vi "coolUI.vi"(11 "CoolDisplay.lvclass":refnum<class "CoolDisplay.lvclass">) -> ()   [LabVIEW 2018, in "CoolDisplay.lvclass"]
uses:
  CoolDisplay.lvclass
panel:
  out "Waveform Chart":cluster{"Humidity":dbl, "Pressure":dbl}(graph)
  out "Temperature":dbl(slide) scale=0.0..10.0
  out "error out":errorcluster
  in  "error in (no error)":errorcluster
  # "Cool Display"
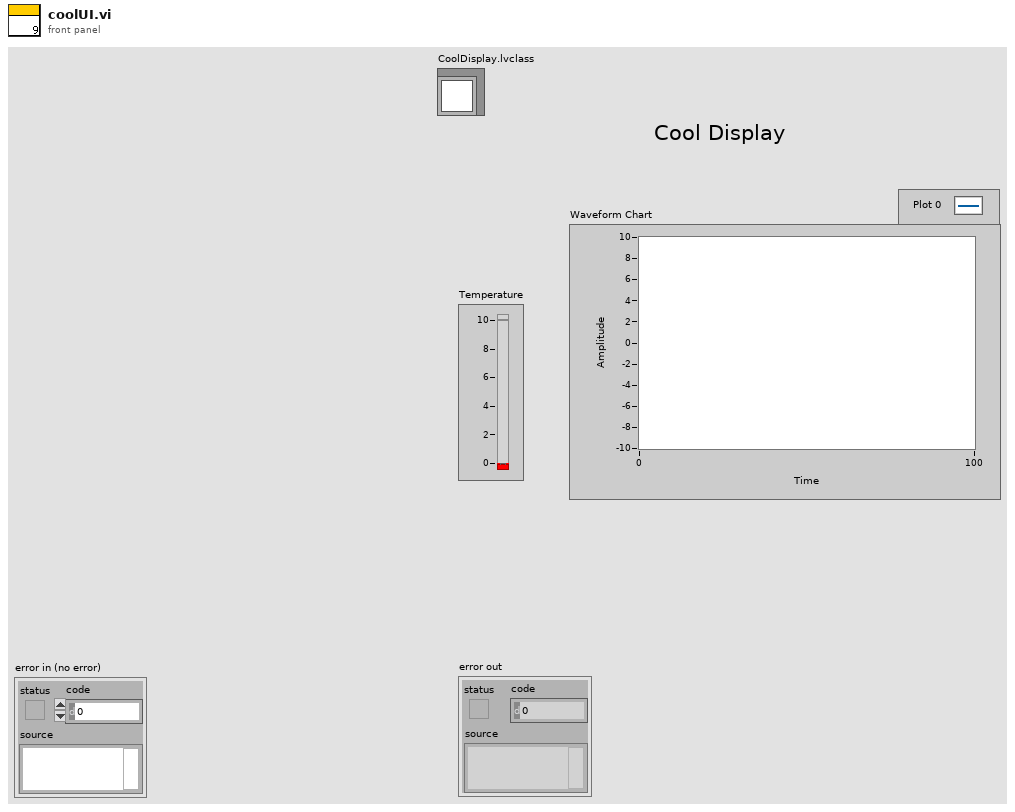
[diagram p1: front panel]
types:
  T1 = enum16{"Always On", "Always Off", "Off While Running"}
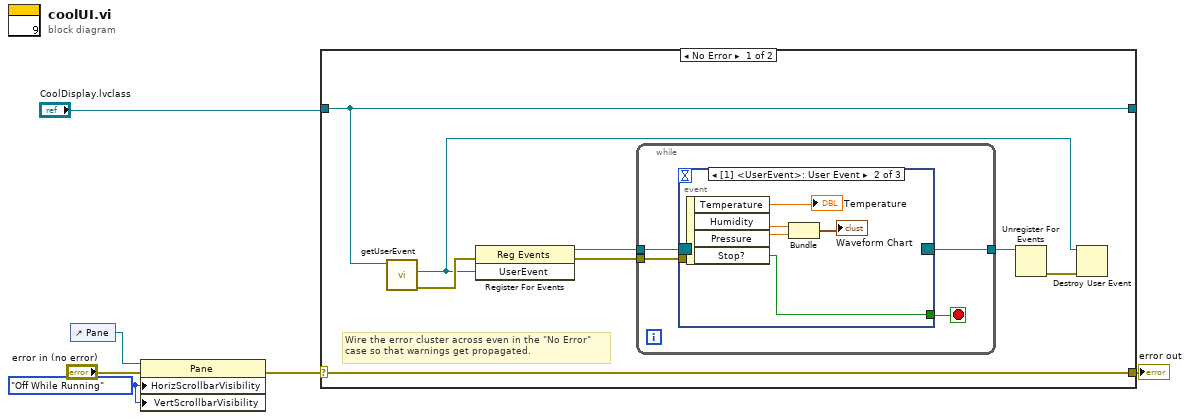
[diagram p0: block diagram]
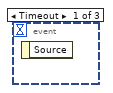
[diagram p2: hidden frame]
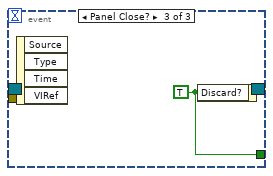
[diagram p3: hidden frame]
diagram:
  w3 = T1."Off While Running" ("Horizontal Scrollbar Visibility")
  n1 = control-ref of="Pane"() -> (w2:refnum<vi>)
  n2 = property class="Pane"(reference=w2, error in="error in (no error)", "HorizScrollbarVisibility"=w3, "VertScrollbarVisibility"=w3) -> (error out=w4:errorcluster)  [unwired: 1 out]
  n3 = case shown="No Error" w4 {
    selector: w4 -> [w14 w26]
    tunnel: [w14 w26] -> w5
    tunnel: [w10 w25] -> _
    tunnel: "CoolDisplay.lvclass" -> [w10 w25]
    frame No Error {
      # "Wire the error cluster across even in the \"No Error\"\ncase so that warnings get propagated."
      n4 = call-dynamic "getUserEvent.vi"("CoolDisplay in"=w10) -> ("error out"=w12:errorcluster, "UserEvent"=w7:refnum<user-event>)  [unwired: 8 in, 1 out]
      n5 = register-events(error in=w12, w7) -> (reference out=w13:refnum<event-registration>, error out=w11:errorcluster)  [unwired: 1 in]
      n6 = while {
        tunnel: w13 -> [w18]
        tunnel: w11 -> [w17]
        tunnel: [w15] -> w9
        stop <- w16 stop-if-true
        n7 = event shown="[1] <UserEvent>: User Event" {
          selector: w18 -> [_ _ _]
          dyn-events: [_ _ _] -> w15
          timeout: _ -> [_ _ _]
          tunnel: w17 -> [_ _ _]
          tunnel: [_ w22 w24] -> w16
          event Timeout {
            n8 = event-data() -> ()  [unwired: 1 in, 1 out]
          }
          event User Event {
            n9 = event-data() -> ("Temperature"=→"Temperature":dbl, "Humidity"=w21:dbl, "Pressure"=w20:dbl, "Stop?"=w22:bool)  [unwired: 1 in]
            n10 = Bundle("Humidity"=w21, "Pressure"=w20) -> (→"Waveform Chart":cluster{"Humidity":dbl, "Pressure":dbl})  [unwired: 1 in]
          }
          event Panel Close? {
            w24 = TRUE ("Discard?")
            n11 = event-data() -> ()  [unwired: 1 in, 4 out]
            n12 = event-data("Discard?"=w24) -> ()  [unwired: 1 in, 1 out]
          }
        }
      }
      n13 = Unregister For Events(event registration refnum=w9) -> (error out=w8:errorcluster)  [unwired: 1 in]
      n14 = Destroy User Event(user event=w7, error in=w8) -> ()  [unwired: 1 out]
    }
    frame Error {
    }
  }
  "error out" <- w5
